vi "MGCC_Commun_OutputChangedSetAnalog (SubVI).vi"(11 "Array in":T1[](array[typedef]) {"value" format="%#_15f"}) -> (1 "Numeric":i32, 3 "Array out":T1[](array[typedef]) {"value" format="%#_15f"})   [LabVIEW 2016]
uses:
  <vilib>/DNP3/DNP3_Master/Analog Info.ctl
  <vilib>/DNP3/DNP3_Master.lvlib
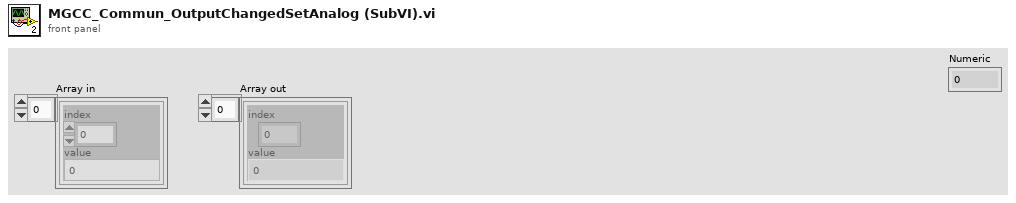
[diagram p1: front panel]
types:
  T1 = typedef "DNP3_Master.lvlib/Analog Info.ctl" = cluster{"index":u16, "value":dbl}
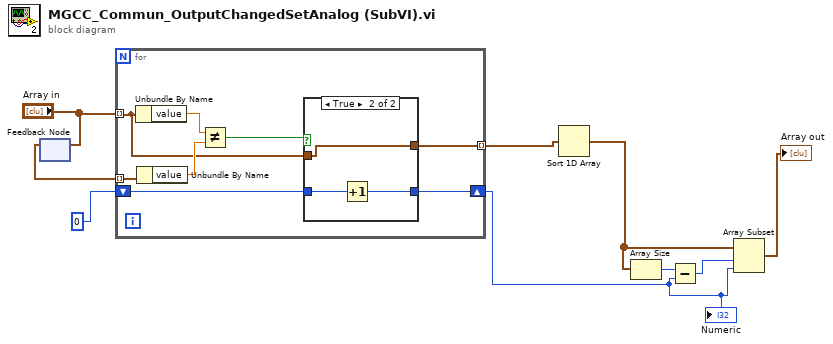
[diagram p0: block diagram]
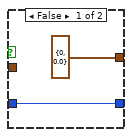
[diagram p2: hidden frame]
diagram:
  n1 = feedback #1() -> (w8:T1[])  [unwired: 1 in]
  n2 = feedback-in #1("Array in") -> ()
  n3 = for {
    tunnel: "Array in" -> [w10] mode=indexing
    tunnel: w8 -> [w17] mode=indexing
    shift-right: [w12] -> w1
    shift-left: 0 -> [w13]
    tunnel: [w11] -> w6 mode=indexing
    n4 = Unbundle By Name(w10) -> ("value"=w16:dbl)
    n5 = Unbundle By Name(w17) -> ("value"=w15:dbl)
    n6 = Not Equal?(x=w16, y=w15) -> (x != y?=w14:bool)
    n7 = case shown="True" w14 {
      tunnel: w13 -> [w18 w22]
      tunnel: [w18 w20] -> w12
      tunnel: [T1 {"index"=0, "value"=0.0} ("f") w21] -> w11
      tunnel: w10 -> [_ w21]
      frame False {
      }
      frame True {
        n8 = Increment(x=w22) -> (x+1=w20:i32)
      }
    }
  }
  "Numeric" <- w1
  n9 = Sort 1D Array(array=w6) -> (sorted array=w4:T1[])
  n10 = Array Size(array=w4) -> (size(s)=w5:i32)
  n11 = Subtract(x=w5, y=w1) -> (x-y=w2:i32)
  n12 = Array Subset(array=w4, index=w2, length=w1) -> (→"Array out":T1[])
